vi "number2frequency.vi"(1 "index(0~31)":i32) -> (0 "Numeric":i32)   [LabVIEW 2014]
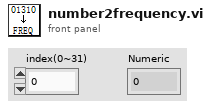
[diagram p1: front panel]
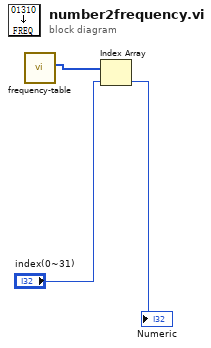
[diagram p0: block diagram]
diagram:
  n1 = call "frequency-table.vi"() -> ("value"=w1:i32[])  [unwired: 11 in]
  n2 = Index Array(array=w1, index="index(0~31)") -> (element=→"Numeric":i32)
